vi "CallTestMethod.vi"(8 "error in":errorcluster, 10 "method":T1, 11 "TestCase in":refnum<class "TestCase.lvclass">) -> (0 "error out":errorcluster, 1 "execution time (sec)":dbl, 2 "Test Method Error":errorcluster, 3 "TestCase out":refnum<class "TestCase.lvclass">)   [LabVIEW 2019, in "TestCase.lvclass"]
uses:
  TestCase.lvclass
  method--Enum.ctl
  TestCase.lvclass/TestCase.ctl
  JKI Reuse/Filter Error Codes (Array)__jki_lib_error_handling -- VI Tester.vi
  JKI Reuse/Filter Error Codes (Scalar)__jki_lib_error_handling -- VI Tester.vi
  Libraries/VITesterUtilities.lvlib
panel:
  # "JKI VI Tester for LabVIEW\nhttp://jkisoft.com/vi-tester\nCopyright (C) 2007-2009, JKI <info@jkisoft.com>\nALL RIGHTS RESERVED"
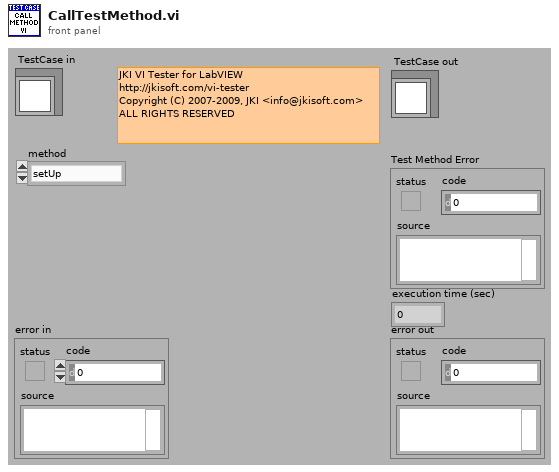
[diagram p1: front panel]
types:
  T1 = typedef "TestCase.lvclass/method--Enum.ctl" = enum16{"setUp", "testMethod", "tearDown"}
  T2 = enum32{"Bad", "Idle", "Run top level", "Running"}
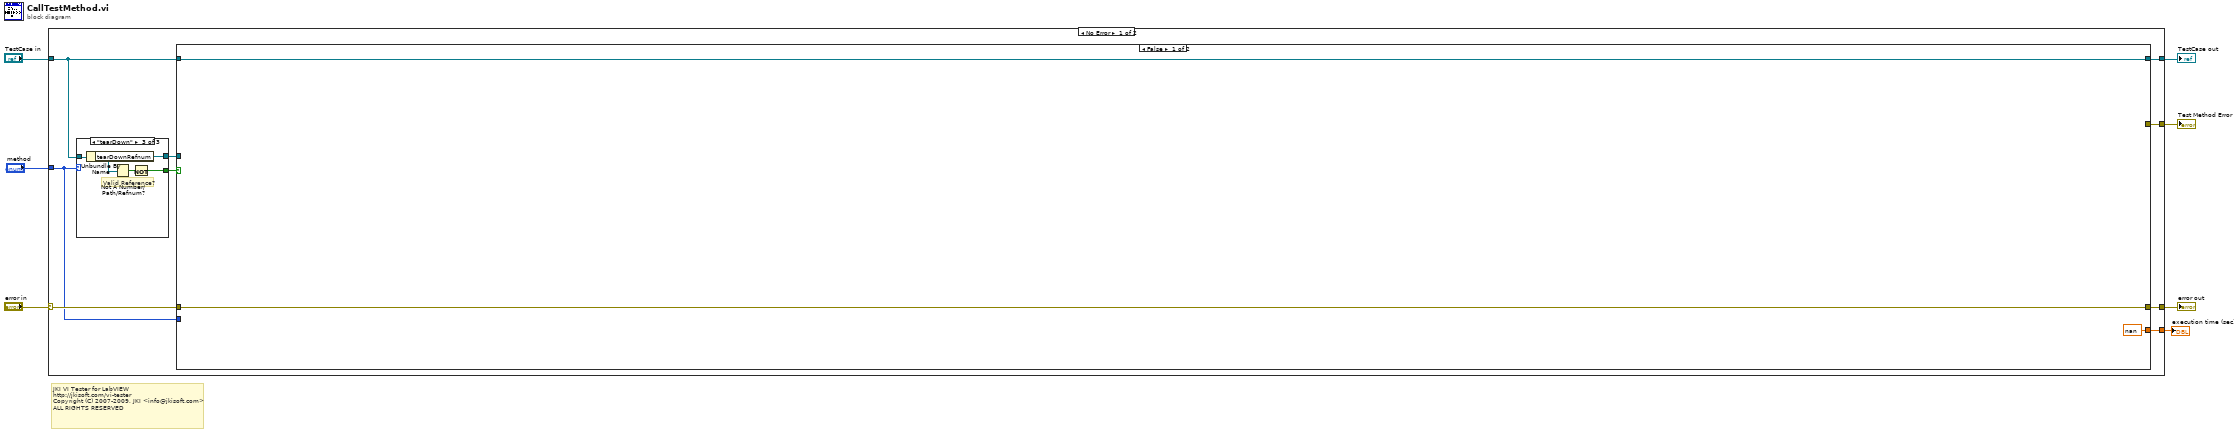
[diagram p0: block diagram]
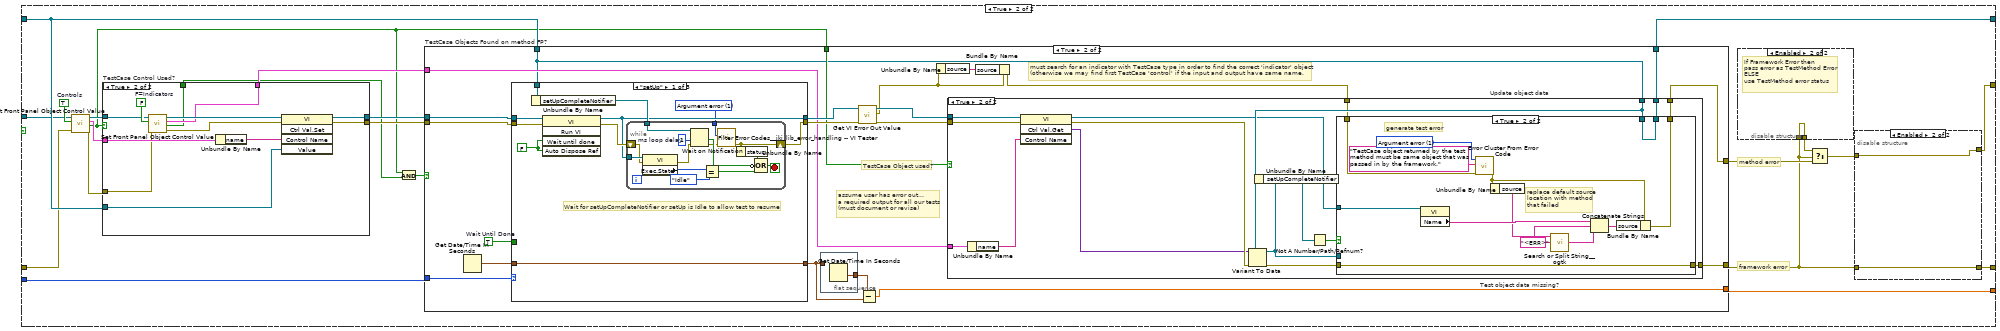
[diagram p2: hidden frame]
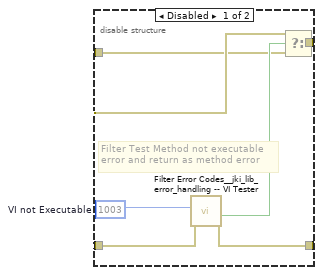
[diagram p3: hidden frame]
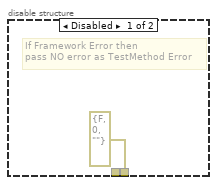
[diagram p4: hidden frame]
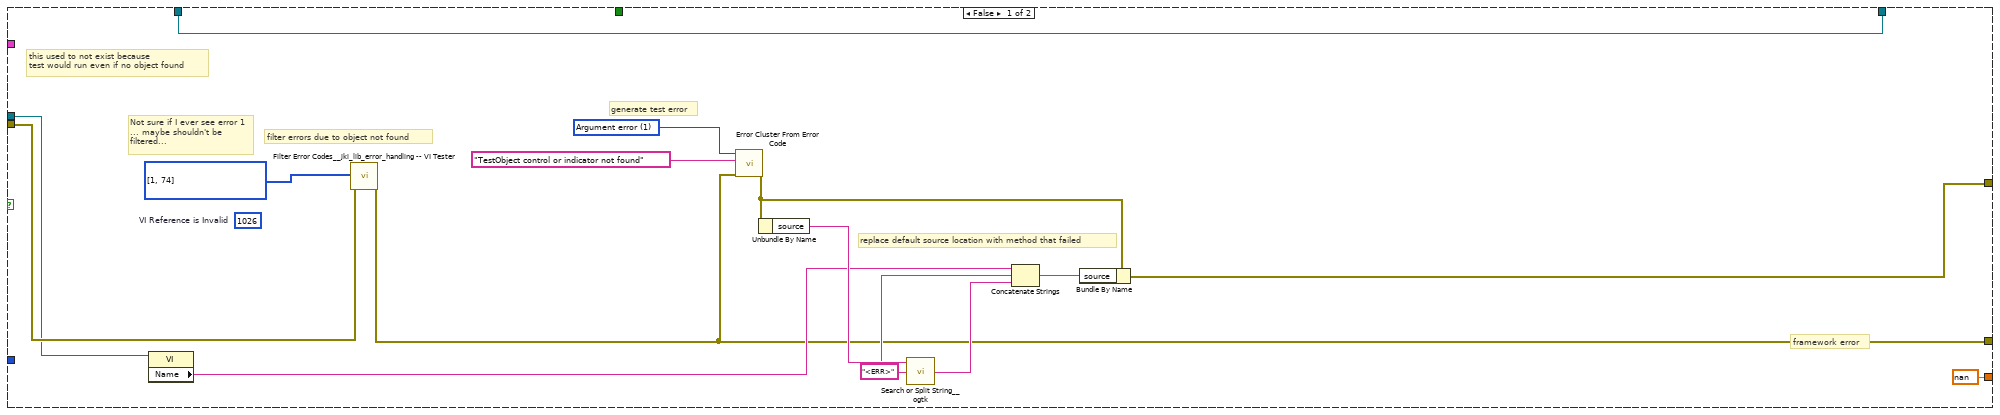
[diagram p5: hidden frame]
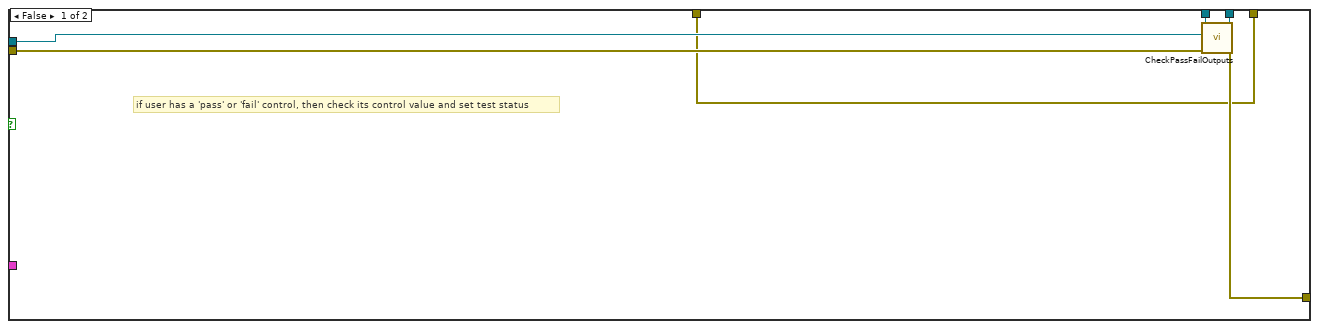
[diagram p6: hidden frame]
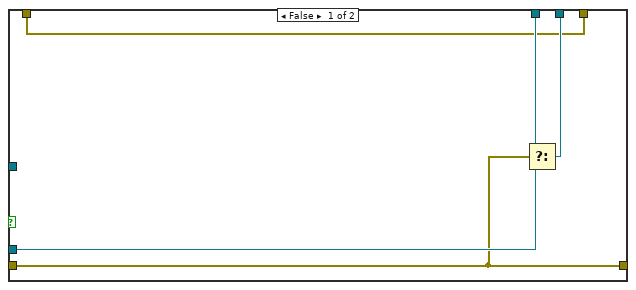
[diagram p7: hidden frame]
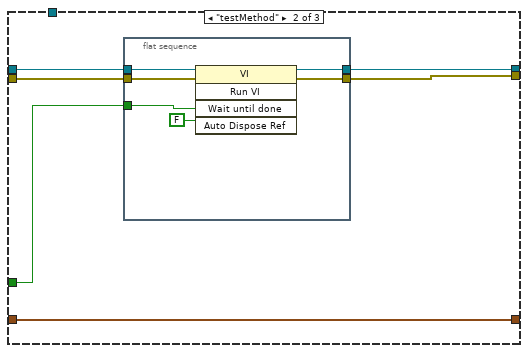
[diagram p8: hidden frame]
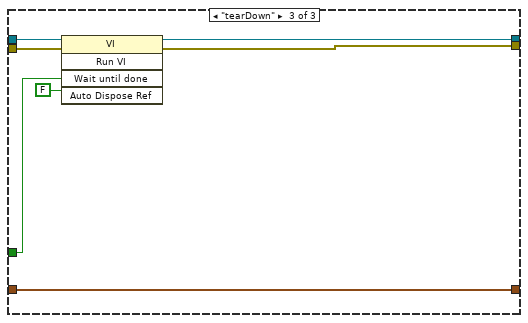
[diagram p9: hidden frame]
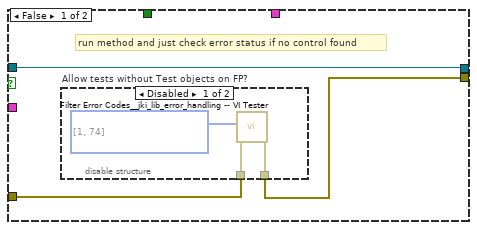
[diagram p10: hidden frame]
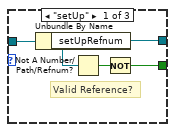
[diagram p12: hidden frame]
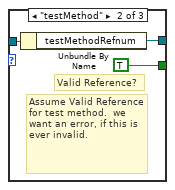
[diagram p13: hidden frame]
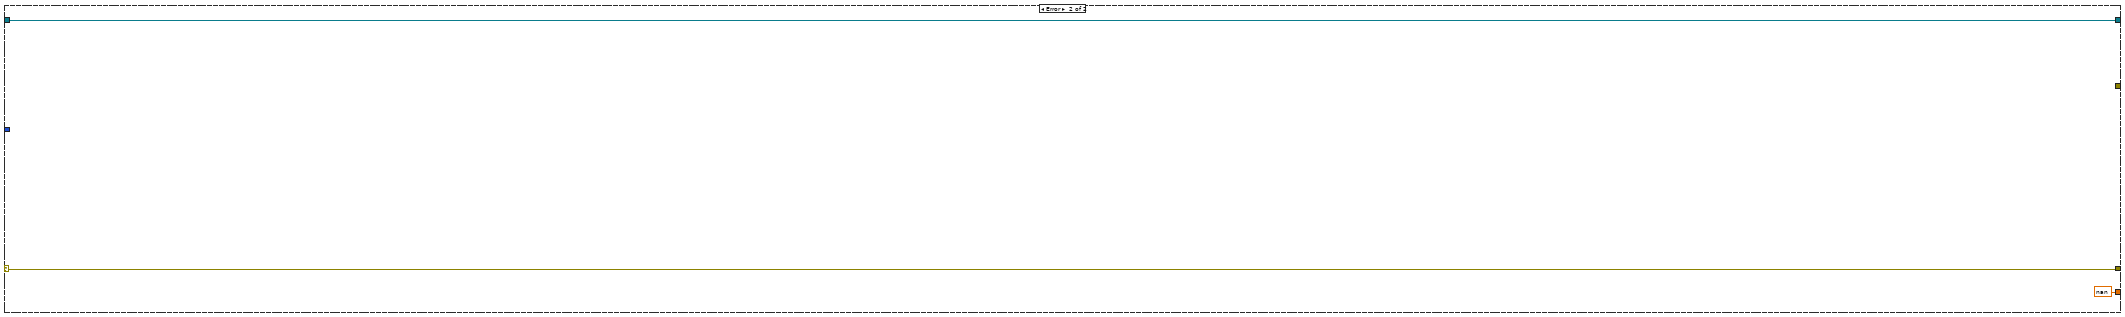
[diagram p14: hidden frame]
diagram:
  # "JKI VI Tester for LabVIEW\nhttp://jkisoft.com/vi-tester\nCopyright (C) 2007-2009, JKI <info@jkisoft.com>\nALL RIGHTS RESERVED"
  n1 = case shown="No Error" "error in" {
    selector: "error in" -> [w11 w204]
    tunnel: [w16 w203] -> w3
    tunnel: [w15 _] -> w4
    tunnel: [w14 w204] -> w5
    tunnel: "TestCase in" -> [w13 w203]
    tunnel: "method" -> [w9 _]
    tunnel: [w8 nan] -> w1
    frame No Error {
      n2 = case shown="\"tearDown\"" w9 {
        tunnel: w13 -> [w194 w197 w201]
        tunnel: [w193 w196 w200] -> w12
        tunnel: [w191 TRUE w198] -> w10
        frame "setUp" {
          # "Valid Reference?"
          n3 = Unbundle By Name(w194) -> ("setUpRefnum"=w193:refnum<vi>)
          n4 = Not A Number/Path/Refnum?(number/path/refnum=w193) -> (NaN/Path/Refnum?=w192:bool)
          n5 = Not(x=w192) -> (.not. x?=w191:bool)
        }
        frame "testMethod" {
          # "Assume Valid Reference for test method.  we want an error, if this is ever invalid."
          # "Valid Reference?"
          n6 = Unbundle By Name(w197) -> ("testMethodRefnum"=w196:refnum<vi>)
        }
        frame "tearDown" {
          # "Valid Reference?"
          n7 = Unbundle By Name(w201) -> ("tearDownRefnum"=w200:refnum<vi>)
          n8 = Not A Number/Path/Refnum?(number/path/refnum=w200) -> (NaN/Path/Refnum?=w199:bool)
          n9 = Not(x=w199) -> (.not. x?=w198:bool)
        }
      }
      n10 = case shown="False" w10 {
        tunnel: [w19 w27] -> w16
        tunnel: [_ w21] -> w15
        tunnel: [w18 w24] -> w14
        tunnel: w13 -> [w19 w36]
        tunnel: w12 -> [_ w32]
        tunnel: w11 -> [w18 w31]
        tunnel: w9 -> [_ w20]
        tunnel: [nan w26] -> w8
        frame False {
        }
        frame True {
          w39 = TRUE  # Controls
          # "method error"
          # "framework error"
          n11 = call "Set Front Panel Object Control Value.vi"("error in"=w31, "Control (F: Indicator)"=w39, "vi reference"=w32) -> ("error out"=w34:errorcluster, "Found?"=w29:bool, "Control Value"=w38:cluster{"name":string, "value":variant}, "dup vi reference"=w37:refnum<vi>)  [unwired: 5 in]
          n12 = case "TestCase Control Used?" shown="True" w29 {
            tunnel: [w172 w190] -> w41
            tunnel: [w173 w189] -> w40
            tunnel: w38 -> [_ w188]
            tunnel: w37 -> [w172 w185]
            tunnel: w36 -> [_ w179]
            tunnel: [_ w181] -> w35
            tunnel: w34 -> [w174 w182]
            tunnel: [_ w180] -> w30
            frame False {
              # "run method and just check error status if no control found"
              n13 = disable-structure "Allow tests without Test objects on FP?" shown="Disabled" {
                disable-tunnel: w174 -> [w177 w178]
                disable-tunnel: [w176 w178] -> w173
                frame Disabled {
                  w175 = i32[] [1, 74] items=["No error", "Argument error", "Memory is full", "Out of zone", "End of file", "File already open", "Generic file I/O error", "File not found", "File permission error", "Disk is full", "Duplicate path", "Too many files open", "System feature not enabled", "Resource file not found", "Cannot add resource", "Resource not found", "Image not found", "Image memory error", "Pen does not exist", "Config type invalid", "Config token not found", "Config parse error", "Config memory error", "Bad external code format", "Bad external code offset", "External code not present", "Null window", "Destroy window error", "Null menu", "Print aborted", "Bad print record", "Print driver error", "Windows error during printing", "Memory error during printing", "Print dialog error", "Generic print error", "Invalid device refnum", "Device not found", "Device parameter error", "Device unit error", "Cannot open device", "Device call aborted", "Generic error", "Cancelled by user", "Object ID too low", "Object ID too high", "Object not in heap", "Unknown heap", "Unknown object (invalid DefProc)", "Unknown object (DefProc not in table)", "Message out of range", "Invalid (null) method", "Unknown message", "Manager call not supported", "Bad address", "Network operation in progress", "Network operation timed out", "Connection is busy", "Network attribute not supported", "Network error", "Address in use", "System out of memory", "Connection aborted", "Connection refused", "Not connected", "Already connected", "Connection closed", "Initialization error (interapplication manager)", "Bad occurrence", "Wait on unbound occurrence handler", "Occurrence queue overflow", "Datalog type conflict", "Unused", "Unrecognized type (interapplication manager)", "Memory corrupt", "Failed to make temporary DLL", "Old CIN version", "Drag socket not found", "Failed to load drop-object", "Failed to register OLE object", "Failed to release OLE object", "Format specifier type mismatch", "Unknown format specifier", "Too few format specifiers", "Too many format specifiers", "Scan failed", "Newer CIN version", "Error converting to variant", "Runtime menu error", "Password tampered", "Variant attribute not found", "Incompatible variant data type", "Event data is not available", "Event Store is not present", "Occurrence is not found", "Event Queue is not created", "Event info is not available", "Refnum passed is NULL", "Error retrieving Class GUID", "Error retrieving CoClass GUID", "Error retrieving TypeLib GUID.", "Bad built application magic bytes.", "Specific driver is different from the specific driver associated with the Logical Name.", "There is no session opened to the class driver.", "Max Error", "MAX - Error with config objects", "MAX - Error loading configuration", "MAX - Group not supported"] ("error codes to filter")
                  n14 = call-poly "Filter Error Codes__jki_lib_error_handling -- VI Tester.vi"("error in"=w177, "error codes to filter"=w175) -> ("error out"=w176:errorcluster)  [unwired: 7 in, 2 out]
                }
                frame Enabled {
                }
              }
            }
            frame True {
              w186 = FALSE  # F=Indicators
              n15 = call "Set Front Panel Object Control Value.vi"("error in"=w182, "Control (F: Indicator)"=w186, "vi reference"=w185) -> ("error out"=w183:errorcluster, "Found?"=w180:bool, "Control Value"=w181:cluster{"name":string, "value":variant}, "dup vi reference"=w184:refnum<vi>)  [unwired: 5 in]
              n16 = Unbundle By Name(w188) -> ("name"=w187:string)
              n17 = invoke class="VI" method="Ctrl Val.Set"(reference=w184, error in=w183, "Control Name"=w187, "Value"=w179) -> (reference out=w190:refnum<vi>, error out=w189:errorcluster)  [unwired: 1 in, 3 out]
            }
          }
          n18 = Compound Arithmetic op=AND(w29, w30) -> (w28:bool)
          n19 = case "TestCase Objects Found on method FP?" shown="True" w28 {
            tunnel: [w63 w87] -> w27
            tunnel: w41 -> [w62 w86]
            tunnel: w40 -> [w66 w85]
            tunnel: w36 -> [w63 w75]
            tunnel: w35 -> [_ w80]
            tunnel: w29 -> [_ w79]
            tunnel: w20 -> [_ w78]
            tunnel: [w54 w73] -> w33
            tunnel: [w56 w76] -> w23
            tunnel: [nan w70] -> w26
            frame False {
              w53 = i32[] [1, 74] items=["No error", "Argument error", "Memory is full", "Out of zone", "End of file", "File already open", "Generic file I/O error", "File not found", "File permission error", "Disk is full", "Duplicate path", "Too many files open", "System feature not enabled", "Resource file not found", "Cannot add resource", "Resource not found", "Image not found", "Image memory error", "Pen does not exist", "Config type invalid", "Config token not found", "Config parse error", "Config memory error", "Bad external code format", "Bad external code offset", "External code not present", "Null window", "Destroy window error", "Null menu", "Print aborted", "Bad print record", "Print driver error", "Windows error during printing", "Memory error during printing", "Print dialog error", "Generic print error", "Invalid device refnum", "Device not found", "Device parameter error", "Device unit error", "Cannot open device", "Device call aborted", "Generic error", "Cancelled by user", "Object ID too low", "Object ID too high", "Object not in heap", "Unknown heap", "Unknown object (invalid DefProc)", "Unknown object (DefProc not in table)", "Message out of range", "Invalid (null) method", "Unknown message", "Manager call not supported", "Bad address", "Network operation in progress", "Network operation timed out", "Connection is busy", "Network attribute not supported", "Network error", "Address in use", "System out of memory", "Connection aborted", "Connection refused", "Not connected", "Already connected", "Connection closed", "Initialization error (interapplication manager)", "Bad occurrence", "Wait on unbound occurrence handler", "Occurrence queue overflow", "Datalog type conflict", "Unused", "Unrecognized type (interapplication manager)", "Memory corrupt", "Failed to make temporary DLL", "Old CIN version", "Drag socket not found", "Failed to load drop-object", "Failed to register OLE object", "Failed to release OLE object", "Format specifier type mismatch", "Unknown format specifier", "Too few format specifiers", "Too many format specifiers", "Scan failed", "Newer CIN version", "Error converting to variant", "Runtime menu error", "Password tampered", "Variant attribute not found", "Incompatible variant data type", "Event data is not available", "Event Store is not present", "Occurrence is not found", "Event Queue is not created", "Event info is not available", "Refnum passed is NULL", "Error retrieving Class GUID", "Error retrieving CoClass GUID", "Error retrieving TypeLib GUID.", "Bad built application magic bytes.", "Specific driver is different from the specific driver associated with the Logical Name.", "There is no session opened to the class driver.", "Max Error", "MAX - Error with config objects", "MAX - Error loading configuration", "MAX - Group not supported"] ("error codes to filter")
              (unwired) 1026  # VI Reference is Invalid
              w59 = "<ERR>" ("search string/char (-)")
              w65 = 1 items=["No error", "Argument error", "Memory is full", "Out of zone", "End of file", "File already open", "Generic file I/O error", "File not found", "File permission error", "Disk is full", "Duplicate path", "Too many files open", "System feature not enabled", "Resource file not found", "Cannot add resource", "Resource not found", "Image not found", "Image memory error", "Pen does not exist", "Config type invalid", "Config token not found", "Config parse error", "Config memory error", "Bad external code format", "Bad external code offset", "External code not present", "Null window", "Destroy window error", "Null menu", "Print aborted", "Bad print record", "Print driver error", "Windows error during printing", "Memory error during printing", "Print dialog error", "Generic print error", "Invalid device refnum", "Device not found", "Device parameter error", "Device unit error", "Cannot open device", "Device call aborted", "Generic error", "Cancelled by user", "Object ID too low", "Object ID too high", "Object not in heap", "Unknown heap", "Unknown object (invalid DefProc)", "Unknown object (DefProc not in table)", "Message out of range", "Invalid (null) method", "Unknown message", "Manager call not supported", "Bad address", "Network operation in progress", "Network operation timed out", "Connection is busy", "Network attribute not supported", "Network error", "Address in use", "System out of memory", "Connection aborted", "Connection refused", "Not connected", "Already connected", "Connection closed", "Initialization error (interapplication manager)", "Bad occurrence", "Wait on unbound occurrence handler", "Occurrence queue overflow", "Datalog type conflict", "Unused", "Unrecognized type (interapplication manager)", "Memory corrupt", "Failed to make temporary DLL", "Old CIN version", "Drag socket not found", "Failed to load drop-object", "Failed to register OLE object", "Failed to release OLE object", "Format specifier type mismatch", "Unknown format specifier", "Too few format specifiers", "Too many format specifiers", "Scan failed", "Newer CIN version", "Error converting to variant", "Runtime menu error", "Password tampered", "Variant attribute not found", "Incompatible variant data type", "Event data is not available", "Event Store is not present", "Occurrence is not found", "Event Queue is not created", "Event info is not available", "Refnum passed is NULL", "Error retrieving Class GUID", "Error retrieving CoClass GUID", "Error retrieving TypeLib GUID.", "Bad built application magic bytes.", "Specific driver is different from the specific driver associated with the Logical Name.", "There is no session opened to the class driver.", "Max Error", "MAX - Error with config objects", "MAX - Error loading configuration", "MAX - Group not supported"]
              # "this used to not exist because\ntest would run even if no object found"
              # "framework error"
              # "generate test error"
              # "Not sure if I ever see error 1 ... maybe shouldn't be filtered..."
              # "filter errors due to object not found"
              # "replace default source location with method that failed"
              n20 = property class="VI"(reference=w62) -> ("Name"=w60:string)  [unwired: 1 in, 2 out]
              n21 = call-poly "Filter Error Codes__jki_lib_error_handling -- VI Tester.vi"("error in"=w66, "error codes to filter"=w53) -> ("error out"=w56:errorcluster)  [unwired: 7 in, 2 out]
              n22 = call <vilib>:"Error Cluster From Error Code.vi"("error in (no error)"=w56, "error message (\"\")"="TestObject control or indicator not found" ("error message (\"\")"), "error code (0)"=w65) -> ("error out"=w55:errorcluster)  [unwired: 6 in]
              n23 = Unbundle By Name(w55) -> ("source"=w61:string)
              n24 = call <userlib>:"Search or Split String__ogtk.vi"("search string/char (-)"=w59, "string"=w61) -> ("substring after match"=w58:string)  [unwired: 1 in, 2 out]
              n25 = Concatenate Strings(w60, w59, w58) -> (w57:string)
              n26 = Bundle By Name(cluster=w55, "source"=w57) -> (w54:errorcluster)
            }
            frame True {
              w81 = TRUE  # Wait Until Done
              # "TestCase Object used?"
              # "must search for an indicator with TestCase type in order to find the correct 'indicator' object\n(otherwise we may find first TestCase 'control' if the input and output have same name."
              # "assume user has error out...\na required output for all our tests\n(must document or revise)"
              n27 = Get Date/Time In Seconds() -> (seconds since 1Jan1904=w72:timestamp)
              n28 = case shown="\"setUp\"" w78 {
                tunnel: w86 -> [w138 w158 w171]
                tunnel: w85 -> [w137 w157 w170]
                tunnel: [w131 w156 w169] -> w84
                tunnel: [w132 w154 w168] -> w83
                tunnel: w81 -> [_ w155 w166]
                tunnel: w75 -> [w135 _ _]
                tunnel: w72 -> [w129 w153 w165]
                tunnel: [w129 w153 w165] -> w69
                frame "setUp" {
                  w130 = 1 items=["No error", "Argument error", "Memory is full", "Out of zone", "End of file", "File already open", "Generic file I/O error", "File not found", "File permission error", "Disk is full", "Duplicate path", "Too many files open", "System feature not enabled", "Resource file not found", "Cannot add resource", "Resource not found", "Image not found", "Image memory error", "Pen does not exist", "Config type invalid", "Config token not found", "Config parse error", "Config memory error", "Bad external code format", "Bad external code offset", "External code not present", "Null window", "Destroy window error", "Null menu", "Print aborted", "Bad print record", "Print driver error", "Windows error during printing", "Memory error during printing", "Print dialog error", "Generic print error", "Invalid device refnum", "Device not found", "Device parameter error", "Device unit error", "Cannot open device", "Device call aborted", "Generic error", "Cancelled by user", "Object ID too low", "Object ID too high", "Object not in heap", "Unknown heap", "Unknown object (invalid DefProc)", "Unknown object (DefProc not in table)", "Message out of range", "Invalid (null) method", "Unknown message", "Manager call not supported", "Bad address", "Network operation in progress", "Network operation timed out", "Connection is busy", "Network attribute not supported", "Network error", "Address in use", "System out of memory", "Connection aborted", "Connection refused", "Not connected", "Already connected", "Connection closed", "Initialization error (interapplication manager)", "Bad occurrence", "Wait on unbound occurrence handler", "Occurrence queue overflow", "Datalog type conflict", "Unused", "Unrecognized type (interapplication manager)", "Memory corrupt", "Failed to make temporary DLL", "Old CIN version", "Drag socket not found", "Failed to load drop-object", "Failed to register OLE object", "Failed to release OLE object", "Format specifier type mismatch", "Unknown format specifier", "Too few format specifiers", "Too many format specifiers", "Scan failed", "Newer CIN version", "Error converting to variant", "Runtime menu error", "Password tampered", "Variant attribute not found", "Incompatible variant data type", "Event data is not available", "Event Store is not present", "Occurrence is not found", "Event Queue is not created", "Event info is not available", "Refnum passed is NULL", "Error retrieving Class GUID", "Error retrieving CoClass GUID", "Error retrieving TypeLib GUID.", "Bad built application magic bytes.", "Specific driver is different from the specific driver associated with the Logical Name.", "There is no session opened to the class driver.", "Max Error", "MAX - Error with config objects", "MAX - Error loading configuration", "MAX - Group not supported"]
                  w136 = FALSE ("Auto Dispose Reference")
                  # "Wait for setUpCompleteNotifier or setUp is Idle to allow test to resume"
                  n29 = Unbundle By Name(w135) -> ("setUpCompleteNotifier"=w134:refnum<notifier>)
                  n30 = invoke class="VI" method="Run VI"(reference=w138, error in=w137, "Wait until done"=w136, "Auto Dispose Ref"=w136) -> (reference out=w131:refnum<vi>, error out=w133:errorcluster)  [unwired: 1 in, 3 out]
                  n31 = while {
                    tunnel: w134 -> [w152]
                    tunnel: w131 -> [w150]
                    shift-right: [w140] -> w132
                    shift-left: w133 -> [w149]
                    tunnel: w130 -> [w139]
                    stop <- w142 stop-if-true
                    w151 = 1  # ms loop delay
                    n32 = property class="VI"(reference=w150, error in=w149) -> (error out=w148:errorcluster, "Exec.State"=w147:T2)  [unwired: 1 out]
                    n33 = Wait on Notification(notifier=w152, timeout in ms (-1)=w151, error in (no error)=w148) -> (timed out?=w144:bool, error out=w141:errorcluster)  [unwired: 1 in, 2 out]
                    n34 = Equal?(x=w147, y=T2."Idle") -> (x = y?=w145:bool)
                    n35 = call-poly "Filter Error Codes__jki_lib_error_handling -- VI Tester.vi"("error in"=w141, "error code to filter"=w139) -> ("error out"=w140:errorcluster)  [unwired: 7 in, 2 out]
                    n36 = Unbundle By Name(w140) -> ("status"=w143:bool)
                    n37 = Compound Arithmetic op=OR(w143, invert w144, w145) -> (w142:bool)
                  }
                }
                frame "testMethod" {
                  n38 = flat-sequence {
                    tunnel: w158 -> [w164]
                    tunnel: w157 -> [w163]
                    tunnel: [w162] -> w156
                    tunnel: [w161] -> w154
                    tunnel: w155 -> [w159]
                    frame #0 {
                      n39 = invoke class="VI" method="Run VI"(reference=w164, error in=w163, "Wait until done"=w159, "Auto Dispose Ref"=FALSE ("Auto Dispose Reference")) -> (reference out=w162:refnum<vi>, error out=w161:errorcluster)  [unwired: 1 in, 3 out]
                    }
                  }
                }
                frame "tearDown" {
                  n40 = invoke class="VI" method="Run VI"(reference=w171, error in=w170, "Wait until done"=w166, "Auto Dispose Ref"=FALSE ("Auto Dispose Reference")) -> (reference out=w169:refnum<vi>, error out=w168:errorcluster)  [unwired: 1 in, 3 out]
                }
              }
              n41 = flat-sequence {
                tunnel: [w88] -> w71
                tunnel: w69 -> [_]
                frame #0 {
                  n42 = Get Date/Time In Seconds() -> (seconds since 1Jan1904=w88:timestamp)
                }
              }
              n43 = call "Get VI Error Out Value.vi"("error in"=w83, "vi reference in"=w84) -> ("error out"=w68:errorcluster, "vi error out"=w67:errorcluster, "dup vi reference"=w82:refnum<vi>)  [unwired: 7 in]
              n44 = Subtract(x=w71, y=w69) -> (x-y=w70:dbl)
              n45 = Unbundle By Name(w67) -> ("source"=w77:string)
              n46 = Bundle By Name(cluster=w67, "source"=w77) -> (w74:errorcluster)
              n47 = case "Update object data" shown="True" w79 {
                tunnel: [w91 w110] -> w87
                tunnel: w82 -> [w90 w109]
                tunnel: w68 -> [w94 w108]
                tunnel: w75 -> [w92 w107]
                tunnel: [w93 w100] -> w76
                tunnel: w80 -> [_ w104]
                tunnel: w74 -> [w89 w98]
                tunnel: [w89 w97] -> w73
                frame False {
                  # "if user has a 'pass' or 'fail' control, then check its control value and set test status"
                  n48 = call "CheckPassFailOutputs.vi"("error in"=w94, "test vi reference"=w90, "TestCase in"=w92) -> ("error out"=w93:errorcluster, "TestCase out"=w91:refnum<class "TestCase.lvclass">)  [unwired: 7 in]
                }
                frame True {
                  n49 = Unbundle By Name(w104) -> ("name"=w96:string)
                  n50 = invoke class="VI" method="Ctrl Val.Get"(reference=w109, error in=w108, "Control Name"=w96) -> (reference out=w99:refnum<vi>, error out=w106:errorcluster, "Get Control Value Variant"=w95:variant)  [unwired: 1 in, 1 out]
                  n51 = Variant To Data(error in=w106, type=w107, Variant=w95) -> (data=w103:refnum<class "TestCase.lvclass">, error out=w105:errorcluster)
                  n52 = Unbundle By Name(w103) -> ("setUpCompleteNotifier"=w102:refnum<notifier>)
                  n53 = Not A Number/Path/Refnum?(number/path/refnum=w102) -> (NaN/Path/Refnum?=w101:bool)
                  n54 = case "Test object data missing?" shown="True" w101 {
                    tunnel: [w115 w128] -> w110
                    tunnel: w107 -> [w114 w128]
                    tunnel: w105 -> [w112 w118]
                    tunnel: w103 -> [w113 _]
                    tunnel: [w112 w118] -> w100
                    tunnel: w99 -> [_ w119]
                    tunnel: w98 -> [w111 w117]
                    tunnel: [w111 w116] -> w97
                    frame False {
                      n55 = Select(t=w114, s=w112, f=w113) -> (s? t:f=w115:refnum<class "TestCase.lvclass">)
                    }
                    frame True {
                      w123 = "<ERR>" ("search string/char (-)")
                      w126 = 1 items=["No error", "Argument error", "Memory is full", "Out of zone", "End of file", "File already open", "Generic file I/O error", "File not found", "File permission error", "Disk is full", "Duplicate path", "Too many files open", "System feature not enabled", "Resource file not found", "Cannot add resource", "Resource not found", "Image not found", "Image memory error", "Pen does not exist", "Config type invalid", "Config token not found", "Config parse error", "Config memory error", "Bad external code format", "Bad external code offset", "External code not present", "Null window", "Destroy window error", "Null menu", "Print aborted", "Bad print record", "Print driver error", "Windows error during printing", "Memory error during printing", "Print dialog error", "Generic print error", "Invalid device refnum", "Device not found", "Device parameter error", "Device unit error", "Cannot open device", "Device call aborted", "Generic error", "Cancelled by user", "Object ID too low", "Object ID too high", "Object not in heap", "Unknown heap", "Unknown object (invalid DefProc)", "Unknown object (DefProc not in table)", "Message out of range", "Invalid (null) method", "Unknown message", "Manager call not supported", "Bad address", "Network operation in progress", "Network operation timed out", "Connection is busy", "Network attribute not supported", "Network error", "Address in use", "System out of memory", "Connection aborted", "Connection refused", "Not connected", "Already connected", "Connection closed", "Initialization error (interapplication manager)", "Bad occurrence", "Wait on unbound occurrence handler", "Occurrence queue overflow", "Datalog type conflict", "Unused", "Unrecognized type (interapplication manager)", "Memory corrupt", "Failed to make temporary DLL", "Old CIN version", "Drag socket not found", "Failed to load drop-object", "Failed to register OLE object", "Failed to release OLE object", "Format specifier type mismatch", "Unknown format specifier", "Too few format specifiers", "Too many format specifiers", "Scan failed", "Newer CIN version", "Error converting to variant", "Runtime menu error", "Password tampered", "Variant attribute not found", "Incompatible variant data type", "Event data is not available", "Event Store is not present", "Occurrence is not found", "Event Queue is not created", "Event info is not available", "Refnum passed is NULL", "Error retrieving Class GUID", "Error retrieving CoClass GUID", "Error retrieving TypeLib GUID.", "Bad built application magic bytes.", "Specific driver is different from the specific driver associated with the Logical Name.", "There is no session opened to the class driver.", "Max Error", "MAX - Error with config objects", "MAX - Error loading configuration", "MAX - Group not supported"]
                      # "generate test error"
                      # "replace default source location with method that failed"
                      n56 = property class="VI"(reference=w119) -> ("Name"=w127:string)  [unwired: 1 in, 2 out]
                      n57 = call <vilib>:"Error Cluster From Error Code.vi"("error in (no error)"=w117, "error message (\"\")"="TestCase object returned by the test method must be same object that was passed in by the framework." ("error message (\"\")"), "error code (0)"=w126) -> ("error out"=w120:errorcluster)  [unwired: 6 in]
                      n58 = Unbundle By Name(w120) -> ("source"=w124:string)
                      n59 = call <userlib>:"Search or Split String__ogtk.vi"("search string/char (-)"=w123, "string"=w124) -> ("substring after match"=w122:string)  [unwired: 1 in, 2 out]
                      n60 = Concatenate Strings(w127, w123, w122) -> (w121:string)
                      n61 = Bundle By Name(cluster=w120, "source"=w121) -> (w116:errorcluster)
                    }
                  }
                }
              }
            }
          }
          n62 = disable-structure shown="Enabled" {
            disable-tunnel: [errorcluster {"status"=FALSE, "code"=0, "source"=""} ("t") w51] -> w25
            disable-tunnel: w23 -> [_ w51]
            frame Disabled {
              # "If Framework Error then\npass NO error as TestMethod Error"
            }
            frame Enabled {
              # "If Framework Error then\npass error as TestMethod Error\nELSE\nuse TestMethod error status"
            }
          }
          n63 = Select(t=w25, s=w23, f=w33) -> (s? t:f=w22:errorcluster)
          n64 = disable-structure shown="Enabled" {
            disable-tunnel: [w46 w48] -> w24
            disable-tunnel: w23 -> [w44 w48]
            disable-tunnel: w22 -> [w43 w49]
            disable-tunnel: [w42 w49] -> w21
            frame Disabled {
              w47 = 1003  # VI not Executable
              # "Filter Test Method not executable\nerror and return as method error"
              n65 = call-poly "Filter Error Codes__jki_lib_error_handling -- VI Tester.vi"("error in"=w44, "error code to filter"=w47) -> ("error out"=w46:errorcluster, "error filtered?"=w45:bool)  [unwired: 7 in, 1 out]
              n66 = Select(t=w44, s=w45, f=w43) -> (s? t:f=w42:errorcluster)
            }
            frame Enabled {
            }
          }
        }
      }
    }
    frame Error {
    }
  }
  "error out" <- w5
  "Test Method Error" <- w4
  "TestCase out" <- w3
  "execution time (sec)" <- w1
